vi "Signal Generator.vi"(1 "Signal Properties":T1={"Schedule"=enum."Constant", "Value"=0.0, "Start Value"=0.0, "End Value"=0.0, "Min Value"=0.0, "Max Value"=0.0, "Duty Cycle (%)"=0.0, "Signal Type"=enum."Sine Wave", "Cycle Number"=0.0, "Phase (degrees)"=0.0, "formula"="1*(step(170-t)*cos(0.62831853071*t)+step(t-170)*cos(0.62831853071*(t-170))*(-1))", "formula length (nm)"=340.0, "formula resolution (nm)"=0.001}, 2 "Points":cluster{"X":dbl, "Y":dbl}[](array[cluster])) -> (0 "Signal":dbl[](array[numeric]))   [LabVIEW 2016]
uses:
  typedefs/Voltage - cluster.ctl
  typedefs/Schedule - enum.ctl
  typedefs/Signal Type - enum.ctl
  <vilib>/measure/NI_MABase.lvlib
  <vilib>/gmath/NI_Gmath.lvlib
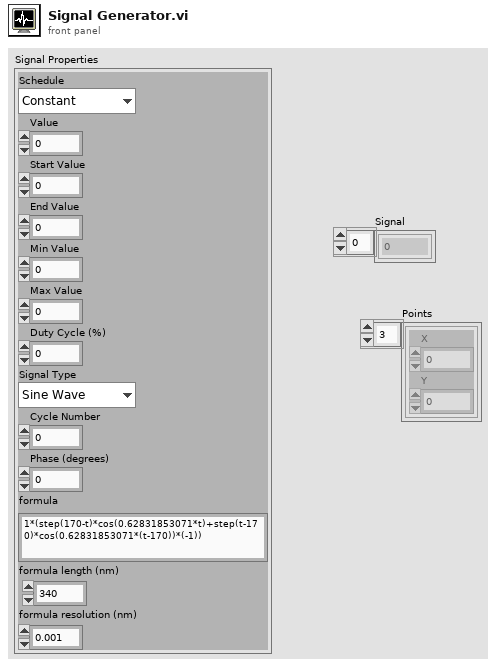
[diagram p1: front panel]
types:
  T1 = typedef "Voltage - cluster.ctl" = cluster{"Schedule":T2, "Value":dbl, "Start Value":dbl, "End Value":dbl, "Min Value":dbl, "Max Value":dbl, "Duty Cycle (%)":dbl, "Signal Type":T3, "Cycle Number":dbl, "Phase (degrees)":dbl, "formula":string, "formula length (nm)":dbl, "formula resolution (nm)":dbl}
  T2 = typedef "Schedule - enum.ctl" = enum16{"Constant", "Ramp", "Fn. Generator", "Formula"}
  T3 = typedef "Signal Type - enum.ctl" = enum16{"Sine Wave", "Triangle Wave", "Square Wave", "Sawtooth Wave"}
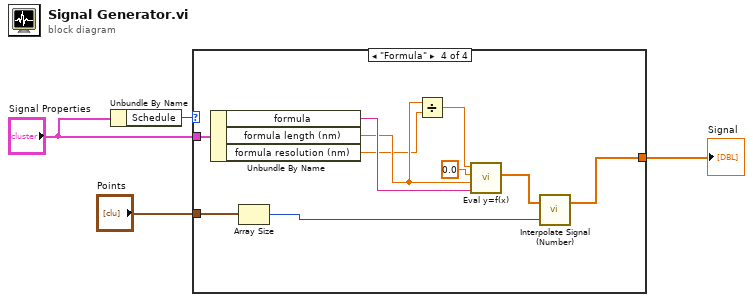
[diagram p0: block diagram]
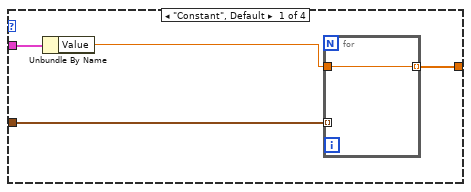
[diagram p2: hidden frame]
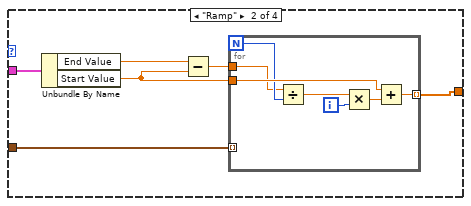
[diagram p3: hidden frame]
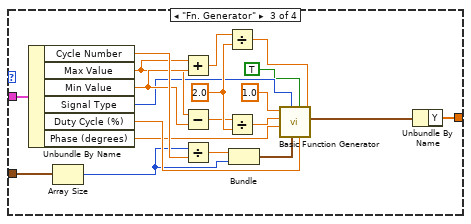
[diagram p4: hidden frame]
diagram:
  n1 = Unbundle By Name("Signal Properties") -> ("Schedule"=w3:T2)
  n2 = case shown="\"Formula\"" w3 {
    tunnel: "Signal Properties" -> [w8 w14 w42 w52]
    tunnel: "Points" -> [w7 w15 w26 w47]
    tunnel: [w5 w10 w41 w44] -> w4
    frame "Constant", Default {
      n3 = Unbundle By Name(w8) -> ("Value"=w6:dbl)
      n4 = for {
        tunnel: w7 -> [_] mode=indexing
        tunnel: w6 -> [w9]
        tunnel: [w9] -> w5 mode=indexing
      }
    }
    frame "Ramp" {
      n5 = Unbundle By Name(w14) -> ("End Value"=w13:dbl, "Start Value"=w11:dbl)
      n6 = Subtract(x=w13, y=w11) -> (x-y=w12:dbl)
      n7 = for {
        N -> [w17]
        tunnel: w15 -> [_] mode=indexing
        tunnel: w12 -> [w16]
        tunnel: w11 -> [w20]
        tunnel: [w19] -> w10 mode=indexing
        i -> [w22]
        n8 = Divide(x=w16, y=w17) -> (x/y=w18:dbl)
        n9 = Multiply(x=w18, y=w22) -> (x*y=w21:dbl)
        n10 = Add(x=w20, y=w21) -> (x+y=w19:dbl)
      }
    }
    frame "Fn. Generator" {
      w36 = 2.0 ("y")
      n11 = Unbundle By Name(w42) -> ("Cycle Number"=w39:dbl, "Max Value"=w33:dbl, "Min Value"=w34:dbl, "Signal Type"=w32:T3, "Duty Cycle (%)"=w38:dbl, "Phase (degrees)"=w27:dbl)
      n12 = Array Size(array=w26) -> (size(s)=w25:i32)
      n13 = Add(x=w33, y=w34) -> (x+y=w30:dbl)
      n14 = Subtract(x=w33, y=w34) -> (x-y=w35:dbl)
      n15 = Divide(x=w25, y=w39) -> (x/y=w40:dbl)
      n16 = Divide(x=w30, y=w36) -> (x/y=w31:dbl)
      n17 = Divide(x=w35, y=w36) -> (x/y=w37:dbl)
      n18 = Bundle(w40, w25) -> (w24:cluster{dbl, i32})  [unwired: 1 in]
      n19 = call <vilib>:"Basic Function Generator.vi"("offset"=w31, "square wave duty cycle (%)"=w38, "reset signal"=TRUE, "sampling info"=w24, "signal type"=w32, "phase"=w27, "amplitude"=w37, "frequency"=1.0) -> ("signal out"=w28:waveform(dbl))  [unwired: 1 in, 2 out]
      n20 = Unbundle By Name(w28) -> ("Y"=w41:dbl[])
    }
    frame "Formula" {
      n21 = Unbundle By Name(w52) -> ("formula"=w50:string, "formula length (nm)"=w49:dbl, "formula resolution (nm)"=w48:dbl)
      n22 = Array Size(array=w47) -> (size(s)=w43:i32)
      n23 = Divide(x=w49, y=w48) -> (x/y=w46:dbl)
      n24 = call <vilib>:"Eval y=f(x).vi"("formula"=w50, "end"=w49, "start"=0.0, "number of points"=w46) -> ("Y Values"=w45:dbl[])  [unwired: 3 out]
      n25 = call "Interpolate Signal (Number).vi"("desired # of points"=w43, "Array"=w45) -> ("Resampled Array"=w44:dbl[])  [unwired: 1 in]
    }
  }
  "Signal" <- w4
